vi "PV Fehler.vi"(9 "error in":errorcluster caption="Fehler", 10 "Istwerte":u16[](array[numeric])) -> (1 "error out":errorcluster caption="Fehler")   [LabVIEW 2020, in "PNS.lvlib"]
uses:
  PNS.lvlib
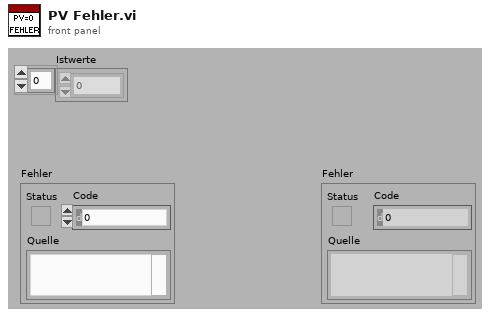
[diagram p1: front panel]
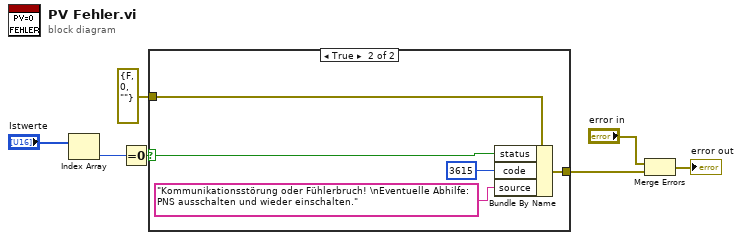
[diagram p0: block diagram]
diagram:
  n1 = Index Array(array="Istwerte") -> (element=w6:u16)  [unwired: 1 in]
  n2 = Equal To 0?(x=w6) -> (x = 0?=w1:bool)
  n3 = case shown="True" w1 {
    selector: w1 -> [_ w9]
    tunnel: errorcluster {"status"=FALSE, "code"=0, "source"=""} ("error out") -> [w8 w13]
    tunnel: [w8 w10] -> w3
    frame False {
    }
    frame True {
      n4 = Bundle By Name(cluster=w13, "status"=w9, "code"=3615, "source"="Kommunikationsstörung oder Fühlerbruch! \nEventuelle Abhilfe: PNS ausschalten und wieder einschalten.") -> (w10:errorcluster)
    }
  }
  n5 = Merge Errors("error in", w3) -> (→"error out":errorcluster)
